vi "Get Data Type Color.vi"(8 "错误输入（无错误）":errorcluster, 11 "数据类型":variant) -> (0 "错误输出":errorcluster, 3 "数据类型颜色":u32(colorbox))   [LabVIEW 2012, in "Application.lvlib"]
uses:
  Application.lvlib
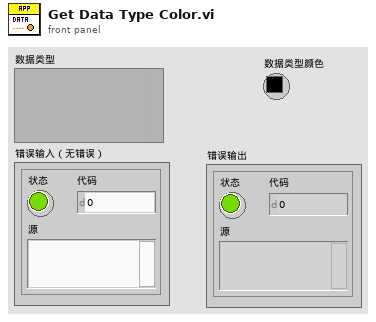
[diagram p1: front panel]
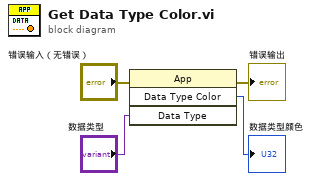
[diagram p0: block diagram]
diagram:
  n1 = invoke class="App" method="Data Type Color"(error in="错误输入（无错误）", "Data Type"="数据类型") -> (error out=→"错误输出":errorcluster, "Data Type Color"=→"数据类型颜色":u32)  [unwired: 2 in, 2 out]
